vi "Emballage_imprimanteParDefaut.vi"(8 "Error in":errorcluster caption="Error in (no error)") -> (0 "Error out":errorcluster, 3 "sous-chaîne suivante":string)   [LabVIEW 2020]
panel:
  out "standard error":string caption="erreur standard"
  out "standard output":string caption="sortie standard"
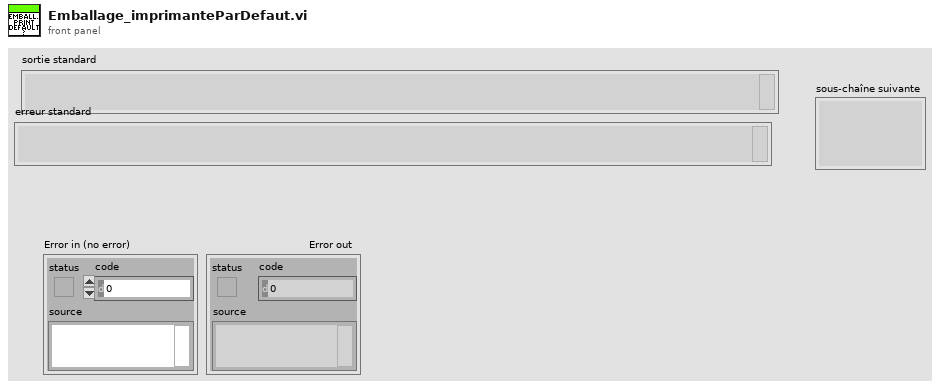
[diagram p1: front panel]
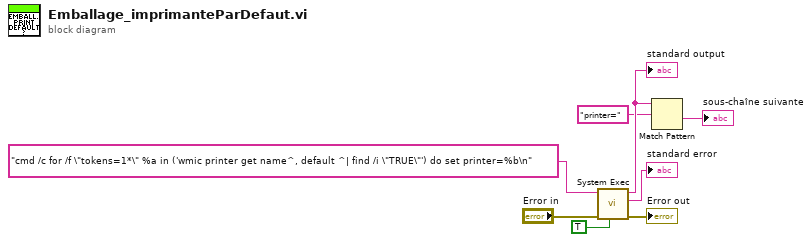
[diagram p0: block diagram]
diagram:
  n1 = call <vilib>:"System Exec.vi"("run minimized? (F)"=TRUE, "error in (no error)"="Error in", "command line"="cmd /c for /f \"tokens=1*\" %a in ('wmic printer get name^, default ^| find /i \"TRUE\"') do set printer=%b\n") -> ("error out"=→"Error out":errorcluster, "standard error"=→"standard error":string, "standard output"=w5:string)  [unwired: 5 in, 1 out]
  "standard output" <- w5
  n2 = Match Pattern(string=w5, regular expression="printer=" ("expression régulière")) -> (after substring=→"sous-chaîne suivante":string)  [unwired: 1 in, 3 out]
